vi "dataAcq_get_interferogram_trace.vi"(0 "reference":refnum<class "OSA.lvclass">, 2 "interferogram trace index":u32, 5 "error in (no error)":errorcluster, 7 "interferogram trace set name":string, 9 "interferogram trace set comment":string) -> (14 "duplicate reference":refnum<class "OSA.lvclass">, 19 "error out":errorcluster)   [LabVIEW 2010, in "OSA.lvclass"]
doc: "Reads data from spectrometer and updates an interferogram trace Y array, X is either equidistant, (x min and max), or a full X-array - call traces_xValueFormat.vi. The trace data buffer is allocated by FTSLib.dll during labview driver initialisation.\n\nX: periods/cm\nY: mW absolute pwr, (pwr/resolution)"
uses:
  OSA.lvclass
  typeDef/trace_properties_string.ctl
  OSA20X_misc.lvlib
  FTSLib.dll
panel:
  in  "parameter":T1=enum."name [max 32]"
  in  "length":u32
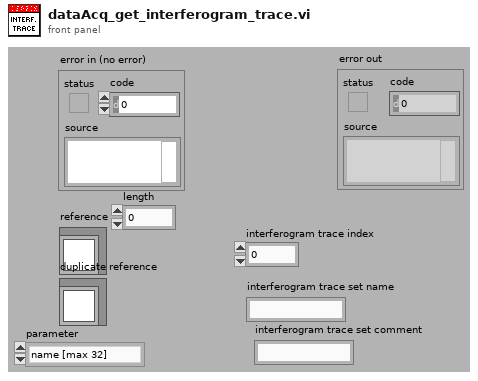
[diagram p1: front panel]
types:
  T1 = typedef "OSA.lvclass/trace_properties_string.ctl" = enum16{"interferometerSerial [max 32]", "name [max 32]", "comment [max 128]", "source [max 24]", "instr_operator [max 24]", "instr_model_str [max 24]", "all_stringParameters"}
  T2 = cluster{"idx":u32, "broadBand":bool, "monoChromatic":bool, "peakToPeakSignal":dbl, "peakToPeakPos":dbl}
  T3 = typedef "OSA.lvclass/ObjectAttributes.ctl" = cluster{"Stop":bool, "dataType":T4, "spectrometerIdx":u16, "buffer size interferogram":i32, "interferogram":cluster{"new":bool, "plot_x_ min":sgl, "plot_x_max":sgl, "plot_y_min":sgl, "plot_y_max":sgl, "Graph Intrfrgrm":T5, "timeStamp":u32, "signal (%)":dbl, "traces":cluster{"idx":u32, "broadBand":bool, "monoChromatic":bool, "peakToPeakSignal":dbl, "peakToPeakPos":dbl}[], "traces idx last":i32}, "spectrum":cluster{"new":bool, "plot_x_min":sgl, "plot_x_max":sgl, "plot_unit_x":T6, "plot_unit_y":T7, "plot_y_min":sgl, "plot_y_max":sgl, "Graph Spectrum":T5, "timeStamp":u32, "X_VAL_OPTIONS":enum16{"MIN_MAX", "ARRAY"}, "traces":cluster{"idx":u32}[], "traces idx last":i32}, "Thorlabs_OSA_64.lvclass:queue_action.ctlqueue ref":refnum<queue>, "action":T8, "plot zoom step":dbl, "buffer semaphore":T9, "acq stopped":bool, "dataType active":T4, "temperature (degr C)":sgl, "pressure (hPa)":sgl, "rel humidity (%)":sgl, "settings":cluster{"resolution":u16, "sensitivity":u16, "Average":bool, "average nr":u32, "apodisation":T10, "acq delay (ms)":u32, "airMesure":T11, "wmtr on":bool, "intfgrm_smooth_width":u16, "intfgrm_smooth_nrOfPasses":u16, "intfgrm_smooth":T12, "phaseCorrection":T13, "zeroFill":u8, "spectr_smooth":T12, "spectr_smooth_width":u16, "spectr_smooth_nrOfPasses":u16, "resolution (/cm)":sgl, "REF wavelength, (nm)":dbl, "gain_idx":u16, "gainAuto":bool, "gain_relative":dbl, "PD sensitivity mode":T14, "PD senseMode implemented":bool, "SensorTemperature implemented":bool, "SensorPressure implemented":bool, "SensorHumidity implemented":bool}, "peaks position":sgl[], "peaks width":sgl[], "peaks height":sgl[], "peaks max nr":u32, "peaks latest nr":i32, "peaks new":bool, "power":dbl, "power new":bool, "path":string, "wavelength (WNr)":dbl, "wavelength new":bool, "buffer size spectrum":i32, "status":string, "VI reference":refnum<vi>, "funcPointer":u64, "libraryPointer":u64, "singleAcquisition":bool, "coherenceLength (cm)":dbl, "coherenceLength new":bool, "spectrometer model":string, "spectrometer serial nr":string, "peaks thld left":sgl[], "peaks thld right":sgl[], "coherenceLength error (cm)":dbl, "ADC bits":u16, "peaks position centroid":sgl[], "peaks height centroid":sgl[], "OSA series":T15, "channel index spectrum":u16, "spectrometer rangeLow, (/cm)":dbl, "spectrometer rangeHigh, (/cm)":dbl, "channel index interferogram":u16}
  T4 = typedef "OSA.lvclass/acq_dataType.ctl" = enum16{"none", "interferogram", "spectrum"}
  T5 = typedef "OSA.lvclass/graph_intensity.ctl" = refnum<vi>
  T6 = typedef "OSA.lvclass/spectrum_x_unit.ctl" = enum16{"wavenr/cm", "THz", "eV", "nm_air", "nm_vac"}
  T7 = typedef "OSA.lvclass/y_unit.ctl" = enum16{"ADC counts", "dBm pwr absolute", "dBm pwr density", "mW pwr absolute", "mW pwr density"}
  T8 = typedef "OSA.lvclass/queue_action.ctl" = enum16{"none", "stop", "GUI_plotInterferogram", "GUI_plotSpectrum", "GUI_plotInterferogramRescale", "GUI_plotSpectrumRescale", "GUI_plotInterferogramReset", "GUI_plotSpectrumReset", "GUI_plotInterferogramAutoScaleY", "GUI_plotSpectrumAutoScaleY", "GUI_plotInterferogramZoomOut", "GUI_plotSpectrumZoomOut", "GUI_plotInterferogramPane", "GUI_plotSpectrumPane", "GUI_plotInterferogramZoomMouse", "GUI_plotSpectrumZoomMouse", "ENVIRONMENT temperature", "ENVIRONMENT pressure", "MODE_resolution set", "MODE_resolution get", "MODE_sensitivity set", "MODE_sensitivity get", "MODE_PDTemperature set", "MODE_PDTemperature get", "REBOOT/RESET firmware", "ACQASYNC_acquireSingleSpectrum", "ACQASYNC_continuous start", "ACQASYNC_continuous stop\n", "ACQASYNC_get last interferogram", "ACQASYNC_get last spectrum", "ACQASYNC_get last waveNr", "ACQOPT_interferogram smoothing set", "ACQOPT_interferogram smoothing get", "ACQOPT_spectrum smoothing set", "ACQOPT_spectrum smoothing get", "ACQOPT_apodisation type set", "ACQOPT_apodisation type get", "ACQOPT_phase correction type set", "ACQOPT_phase correction type get", "ACQOPT_acqIntervall_set", "ACQOPT_acqIntervall_get", "ACQOPT_average spectrum set", "ACQOPT_average spectrum get", "ACQOPT_rolling average set", "ACQOPT_rolling average get", "ACQOPT_zero fill factor set", "ACQOPT_zero fill factor get", "ACQOPT_cycle counting set", "ACQOPT_cycle counting get", "ACQOPT_air measure option set", "ACQOPT_air measure option get", "ACQOPT_gainLevel auto get", "ACQOPT_gainLevel auto set", "ACQOPT_gainLevel get", "ACQOPT_gainLevel set", "ACQOPT_getAll", "INSTRUMENT_PROPERTY_range_WaveNr_min", "INSTRUMENT_PROPERTY_range_WaveNr_max", "INSTRUMENT_PROPERTY_reference_wavelength_cm^-1", "INSTRUMENT_PROPERTY_samplesPerRefPeriod", "INSTRUMENT_PROPERTY_resolution_waveNrPercm", "INSTRUMENT_PROPERTY_availableGainLevels", "INSTRUMENT_PROPERTY_status", "CONVERT", "ANALYSE_POWER", "ANALYSE_PEAKS", "ANALYSE_WAVELENGTH", "ANALYSE_SPECTRUM", "ANALYSE_INTERFEROGRAM", "ANALYSE_COHERENCE_LENGTH", "MATH", "MATH_power", "MATH_peaks", "FILE", "miscellaneous"}
  T9 = typedef "Semaphore RefNum" = refnum<k1>
  T10 = typedef "OSA.lvclass/apodisation.ctl" = enum16{"NONE", "NORTON_BEER_WEAK", "NORTON_BEER_MEDIUM", "NORTON_BEER_STRONG", "TRIANGULAR", "COSINE", "HANN", "HAMMING", "BLACKMANHARRIS3", "BLACKMANHARRIS4", "GAUSSIAN"}
  T11 = typedef "OSA.lvclass/airMeasure.ctl" = enum16{"TEMPERATURE", "PRESSURE"}
  T12 = typedef "OSA20X_misc.lvlib/interferogram_smoothing.ctl" = enum16{"NONE", "BINOMIAL", "SAVITSKY_GOLAY", "FOURIER", "MOVING_AVERAGE", "GAUSSIAN"}
  T13 = typedef "OSA.lvclass/phaseCorrection.ctl" = enum16{"NONE", "MERTZ", "FORMAN", "MERTZ_FILE", "FORMAN_FILE", "FUTURE COMP."}
  T14 = typedef "OSA20X_misc.lvlib/PDTemperatureMode.ctl" = enum16{"cool: better sensitivity/noise floor", "warm: extended wl range"}
  T15 = typedef "OSA.lvclass/OSA_series.ctl" = enum16{"OSA200", "OSA300", "UNKNOWN"}
  T16 = cluster{"idx":u32, "broadBand":bool, "monoChromatic":bool, "peakToPeakSignal":dbl, "peakToPeakPos":dbl}[]
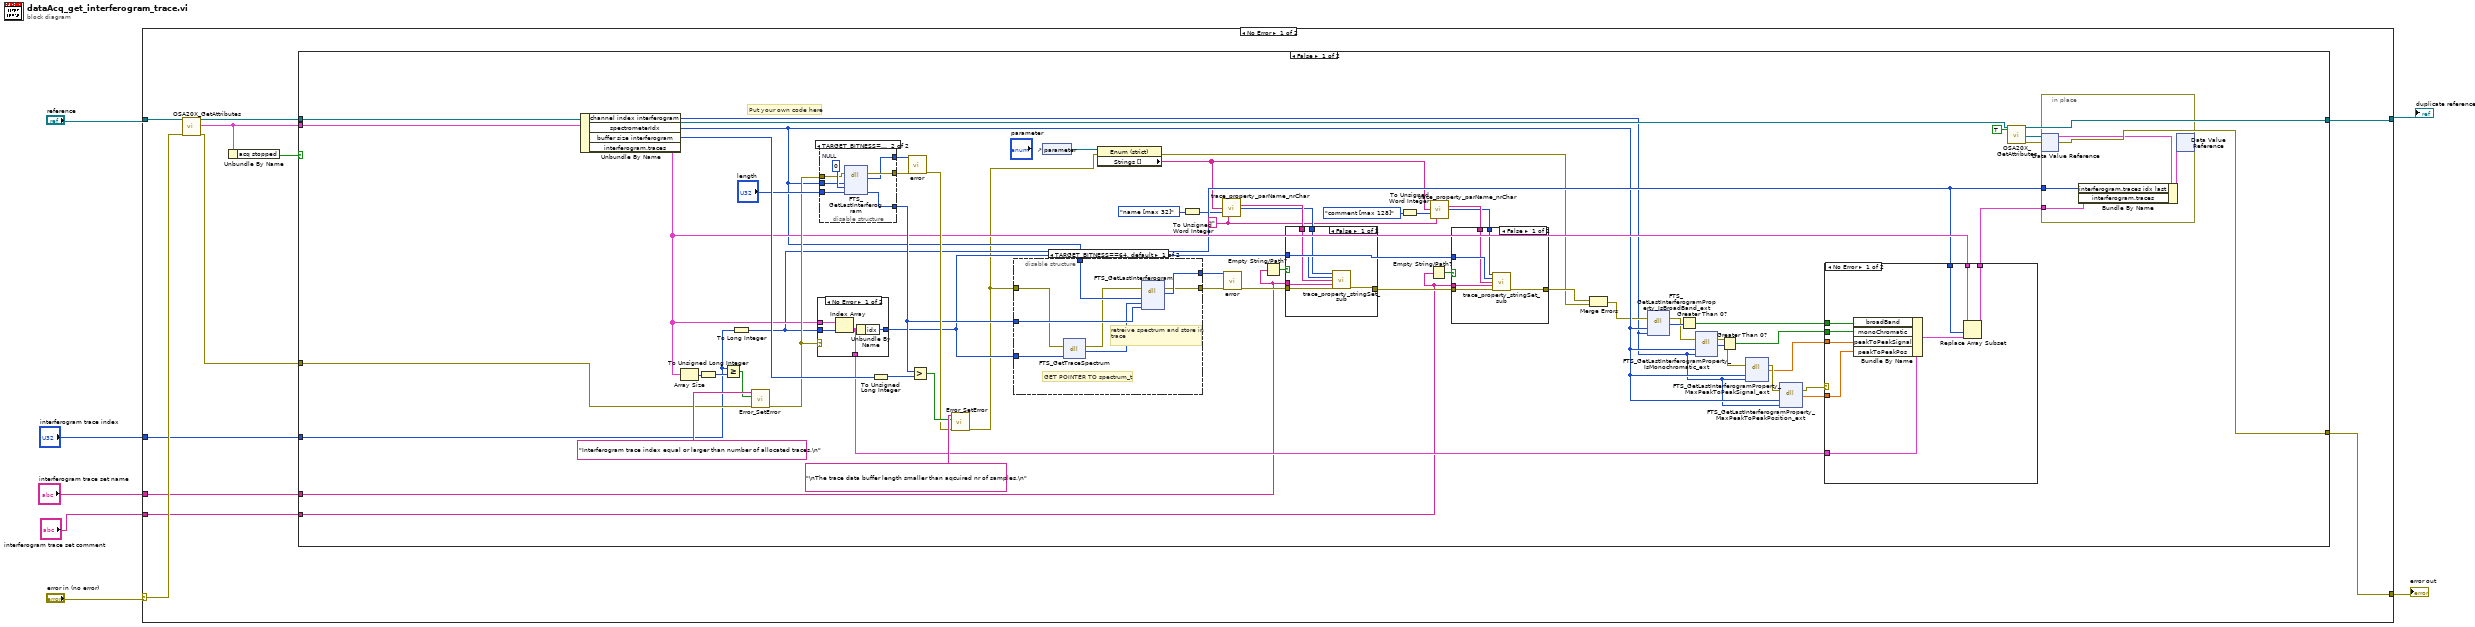
[diagram p0: block diagram]
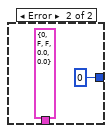
[diagram p5: hidden frame]
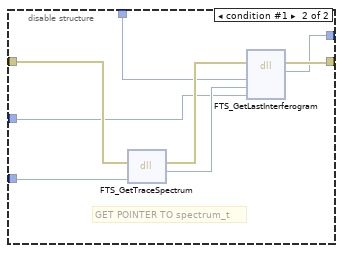
[diagram p6: hidden frame]
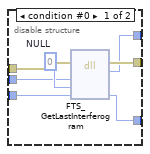
[diagram p7: hidden frame]
diagram:
  n1 = case shown="No Error" "error in (no error)" {
    selector: "error in (no error)" -> [w17 w148]
    tunnel: [w15 w148] -> w6
    tunnel: "reference" -> [w18 w147]
    tunnel: [w16 w147] -> w4
    tunnel: "interferogram trace index" -> [w12 _]
    tunnel: "interferogram trace set name" -> [w9 _]
    tunnel: "interferogram trace set comment" -> [w8 _]
    frame No Error {
      n2 = call "OSA20X_GetAttributes.vi"("reference in"=w18, "error in (no error)"=w17) -> ("reference out"=w14:refnum<class "OSA.lvclass">, "Data"=w13:T3, "error out"=w11:errorcluster)  [unwired: 14 in, 1 out]
      n3 = Unbundle By Name(w13) -> ("acq stopped"=w10:bool)
      n4 = case shown="False" w10 {
        tunnel: w13 -> [w65 _]
        tunnel: w14 -> [w35 w146]
        tunnel: [w77 w146] -> w16
        tunnel: [w76 w145] -> w15
        tunnel: w11 -> [w61 w145]
        tunnel: w12 -> [w43 _]
        tunnel: w9 -> [w38 _]
        tunnel: w8 -> [w37 _]
        frame False {
          w20 = "" ("all string")
          # "Put your own code here"
          n5 = Unbundle By Name(w65) -> ("channel index interferogram"=w19:u16, "spectrometerIdx"=w44:u16, "buffer size interferogram"=w78:i32, "interferogram.traces"=w47:T16)
          n6 = Array Size(array=w47) -> (size(s)=w64:i32)
          n7 = To Unsigned Long Integer(number=w64) -> (unsigned 32bit integer=w63:u32)
          n8 = Greater Or Equal?(x=w43, y=w63) -> (x >= y?=w60:bool)
          n9 = To Long Integer(number=w43) -> (32bit integer=w45:i32)
          n10 = call "Error_SetError.vi"("error in"=w61, "status (true)"=w60, "source(\"\")"="Interferogram trace index equal or larger than number of allocated traces.\n" ("source(\"\")")) -> ("error out"=w59:errorcluster)  [unwired: 4 in]
          n11 = case shown="No Error" w59 {
            tunnel: w47 -> [w108 _]
            tunnel: w45 -> [w107 _]
            tunnel: [w106 u32 0 ("idx")] -> w36
            tunnel: [w105 T2 {"idx"=0, "broadBand"=FALSE, "monoChromatic"=FALSE, "peakToPeakSignal"=0.0, "peakToPeakPos"=0.0} ("Cluster")] -> w53
            frame No Error {
              n12 = Index Array(array=w108, index=w107) -> (element=w105:T2)
              n13 = Unbundle By Name(w105) -> ("idx"=w106:u32)
            }
            frame Error {
            }
          }
          n14 = disable-structure shown="TARGET_BITNESS==64, default" {
            disable-tunnel: w44 -> [w129 w138]
            disable-tunnel: [w127 w135] -> w67
            disable-tunnel: [w133 w139] -> w72
            disable-tunnel: "length" -> [w131 w137]
            disable-tunnel: [w128 w136] -> w70
            disable-tunnel: w59 -> [w132 w134]
            frame condition #0 {
              w130 = u32 0  # NULL
              n15 = dll-call lib="FTSLib.dll" fn="FTS_GetLastInterferogram"(error in=w132, "spectrIdx"=w129, "spec"=w130, "length"=w131) -> (error out=w133:errorcluster, "return type"=w128:i32, "length"=w127:u32)  [unwired: 4 in, 1 out]
            }
            frame condition #1 (active) {
              w140 = u64 0  # NULL
              n16 = dll-call lib="FTSLib.dll" fn="FTS_GetLastInterferogram"(error in=w134, "spectrIdx"=w138, "spec"=w140, "length"=w137) -> (error out=w139:errorcluster, "return type"=w136:i32, "length"=w135:u32)  [unwired: 4 in, 1 out]
            }
          }
          n17 = To Unsigned Long Integer(number=w78) -> (unsigned 32bit integer=w75:u32)
          n18 = call "error.vi"("result code"=w70, "error in (no error)"=w72) -> ("error out"=w71:errorcluster)  [unwired: 15 in, 2 out]
          n19 = Greater?(x=w67, y=w75) -> (0:w79:bool)
          n20 = call "Error_SetError.vi"("error in"=w71, "status (true)"=w79, "source(\"\")"="\nThe trace data buffer length smaller than aqcuired nr of samples.\n" ("source(\"\")")) -> ("error out"=w31:errorcluster)  [unwired: 4 in]
          n21 = disable-structure shown="TARGET_BITNESS==64, default" {
            disable-tunnel: w44 -> [w118 w119]
            disable-tunnel: w31 -> [w113 w123]
            disable-tunnel: [w111 w121] -> w69
            disable-tunnel: [w117 w120] -> w68
            disable-tunnel: w67 -> [w116 w122]
            disable-tunnel: w36 -> [w115 w124]
            frame condition #0 (active) {
              # "retreive spectrum and store in trace"
              # "GET POINTER TO spectrum_t"
              n22 = dll-call lib="FTSLib.dll" fn="FTS_GetTraceSpectrum"(error in=w113, "traceIdx"=w115) -> (error out=w112:errorcluster, "spectrum_t_pointer"=w114:u64)  [unwired: 3 in, 1 out]
              n23 = dll-call lib="FTSLib.dll" fn="FTS_GetLastInterferogram"(error in=w112, "spectrIdx"=w118, "spectrum_t_pointer"=w114, "length"=w116) -> (error out=w111:errorcluster, "return type"=w117:i32)  [unwired: 5 in, 1 out]
            }
            frame condition #1 {
              # "GET POINTER TO spectrum_t"
              n24 = dll-call lib="FTSLib.dll" fn="FTS_GetTraceSpectrum"(error in=w123, "traceIdx"=w124) -> (error out=w125:errorcluster, "spectrum_t_pointer"=w126:u32)  [unwired: 3 in, 1 out]
              n25 = dll-call lib="FTSLib.dll" fn="FTS_GetLastInterferogram"(error in=w125, "spectrIdx"=w119, "spectrum_t_pointer"=w126, "length"=w122) -> (error out=w121:errorcluster, "return type"=w120:i32)  [unwired: 5 in, 1 out]
            }
          }
          n26 = control-ref of="parameter"() -> (w34:refnum<vi>)
          n27 = property class="Enum (strict)"(reference=w34, error in=w31) -> (error out=w29:errorcluster, "Strings []"=w24:string[])  [unwired: 1 out]
          n28 = To Unsigned Word Integer(number=trace_properties_string."name [max 32]" ("parameter")) -> (unsigned 16bit integer=w27:u16)
          n29 = call "trace_property_parName_nrChar.vi"("Strings enum"=w24, "Value enum"=w27, "all string"=w20) -> ("parameter names"=w26:string[], "char nr max"=w25:i32[])  [unwired: 11 in]
          n30 = call "error.vi"("result code"=w68, "error in (no error)"=w69) -> ("error out"=w39:errorcluster)  [unwired: 15 in, 2 out]
          n31 = Empty String/Path?(string/path=w38) -> (empty?=w41:bool)
          n32 = case shown="False" w41 {
            tunnel: [w92 w94] -> w42
            tunnel: w39 -> [w93 w94]
            tunnel: w38 -> [w89 _]
            tunnel: w26 -> [w91 _]
            tunnel: w36 -> [w90 _]
            tunnel: w25 -> [w88 _]
            frame False {
              n33 = call "trace_property_stringSet_sub.vi"("char nr max"=w88, "trace idx global"=w90, "parameter_name"=w91, "parameter_value"=w89, "error in (no error)"=w93) -> ("error out"=w92:errorcluster)  [unwired: 10 in]
            }
            frame True {
            }
          }
          n34 = To Unsigned Word Integer(number=trace_properties_string."comment [max 128]" ("parameter")) -> (unsigned 16bit integer=w23:u16)
          n35 = Empty String/Path?(string/path=w37) -> (empty?=w40:bool)
          n36 = call "trace_property_parName_nrChar.vi"("Strings enum"=w24, "Value enum"=w23, "all string"=w20) -> ("parameter names"=w22:string[], "char nr max"=w21:i32[])  [unwired: 11 in]
          n37 = case shown="False" w40 {
            tunnel: w42 -> [w86 w87]
            tunnel: [w85 w87] -> w30
            tunnel: w37 -> [w83 _]
            tunnel: w36 -> [w84 _]
            tunnel: w22 -> [w82 _]
            tunnel: w21 -> [w81 _]
            frame False {
              n38 = call "trace_property_stringSet_sub.vi"("char nr max"=w81, "trace idx global"=w84, "parameter_name"=w82, "parameter_value"=w83, "error in (no error)"=w86) -> ("error out"=w85:errorcluster)  [unwired: 10 in]
            }
            frame True {
            }
          }
          n39 = Merge Errors(w30, w29) -> (w28:errorcluster)
          n40 = dll-call lib="FTSLib.dll" fn="FTS_GetLastInterferogramProperty_IsBroadBand_ext"(error in=w28, "spectrIdx"=w44, "channel"=w19) -> (error out=w57:errorcluster, "return type"=w58:u8)  [unwired: 4 in, 1 out]
          n41 = Greater Than 0?(x=w58) -> (x > 0?=w52:bool)
          n42 = dll-call lib="FTSLib.dll" fn="FTS_GetLastInterferogramProperty_IsMonochromatic_ext"(error in=w57, "spectrIdx"=w44, "channel"=w19) -> (error out=w54:errorcluster, "return type"=w56:u8)  [unwired: 4 in, 1 out]
          n43 = Greater Than 0?(x=w56) -> (x > 0?=w51:bool)
          n44 = dll-call lib="FTSLib.dll" fn="FTS_GetLastInterferogramProperty_MaxPeakToPeakSignal_ext"(error in=w54, "spectrIdx"=w44, "channel"=w19) -> (error out=w55:errorcluster, "return type"=w50:dbl)  [unwired: 4 in, 1 out]
          n45 = dll-call lib="FTSLib.dll" fn="FTS_GetLastInterferogramProperty_MaxPeakToPeakPosition_ext"(error in=w55, "spectrIdx"=w44, "channel"=w19) -> (error out=w48:errorcluster, "return type"=w49:dbl)  [unwired: 4 in, 1 out]
          n46 = case shown="No Error" w48 {
            tunnel: w53 -> [w103 _]
            tunnel: w52 -> [w102 _]
            tunnel: w51 -> [w101 _]
            tunnel: w50 -> [w100 _]
            tunnel: w49 -> [w99 _]
            tunnel: w47 -> [w98 w104]
            tunnel: [w97 w104] -> w46
            tunnel: w45 -> [w95 _]
            frame No Error {
              n47 = Bundle By Name(cluster=w103, "broadBand"=w102, "monoChromatic"=w101, "peakToPeakSignal"=w100, "peakToPeakPos"=w99) -> (w96:T2)
              n48 = Replace Array Subset(array=w98, new element=w96, index=w95) -> (w97:T16)
            }
            frame Error {
            }
          }
          n49 = call "OSA20X_GetAttributes.vi"("reference in"=w35, "OnlyGetDvrReference(False)"=TRUE) -> ("reference out"=w77:refnum<class "OSA.lvclass">, "DataRef"=w73:refnum<data-value>, "error out"=w76:errorcluster)  [unwired: 14 in, 1 out]
          n50 = in-place {
            in-place-border: w45 -> [w143]
            in-place-border: w46 -> [w141]
            n51 = in-place-dvr #1(w73) -> (w144:T3)  [unwired: 1 out]
            n52 = Bundle By Name(cluster=w144, "interferogram.traces idx last"=w143, "interferogram.traces"=w141) -> (w142:T3)
            n53 = in-place-dvr #1(w142) -> ()  [unwired: 2 out]
          }
        }
        frame True {
        }
      }
    }
    frame Error {
      # "Error"
    }
  }
  "error out" <- w6
  "duplicate reference" <- w4
